vi "get_sensitivity.vi"(8 "input 1":dbl=26.0, 11 "SR850 GPIB In":refnum<visa-resource-name>) -> (0 "error out":errorcluster, 3 "SR850 GPIB Out":refnum<visa-resource-name>)   [LabVIEW 2014]
panel:
  in  "error in":errorcluster
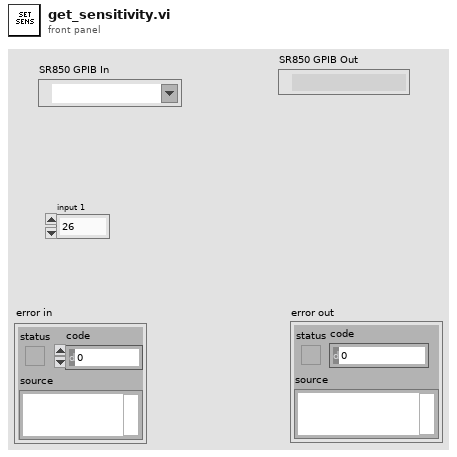
[diagram p1: front panel]
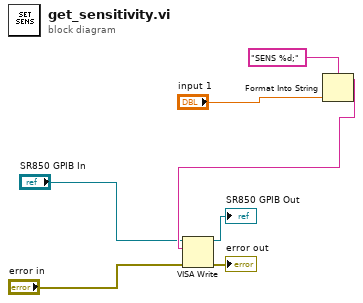
[diagram p0: block diagram]
diagram:
  n1 = Format Into String(format string="SENS %d;", "input 1") -> (resulting string=w4:string)  [unwired: 2 in, 1 out]
  n2 = VISA Write(VISA resource name="SR850 GPIB In", write buffer=w4, error in (no error)="error in") -> (VISA resource name out=→"SR850 GPIB Out":refnum<visa-resource-name>, error out=→"error out":errorcluster)  [unwired: 1 out]
